vi "PH_Cont-601k_PSU.PC Set Interlock.vi"(0 "VI in":refnum<vi>, 2 "Set Interlock":bool, 5 "error in (no error)":errorcluster) -> (14 "VI out":refnum<vi>, 19 "error out":errorcluster)   [LabVIEW 2014, in "PH_Cont-601k_PSU.lvlib"]
uses:
  PH_Cont-601k_PSU.lvlib
  PH_Cont-601k_PSU.Readyness Program.ctl
  PH_Beckhoff/PH_Beckhoff.lvlib
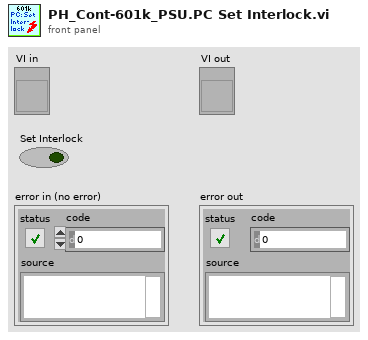
[diagram p1: front panel]
types:
  T1 = typedef "PH_Cont-601k_PSU.lvlib/PH_Cont-601k_PSU.Readyness Program.ctl" = enum32{"OFF", "POWER", "INTERLOCK"}
  T2 = typedef "PH_Cont-601k_PSU.lvlib/PH_Cont-601k_PSU.i attribute.ctl" = cluster{"GUI Refs":T3, "Interlock":bool, "Service ID applied Voltage":i32, "Device Settings":cluster{"Configuration":T4, "Flash Interval [s]":dbl, "Mode":T5, "Voltage [V]":u16, "Charge":bool, "VISA resource name":refnum<visa-resource-name>}, "Readyness":T6, "Information":cluster{"VISA resource name":refnum<visa-resource-name>, "Tagname Power On":string, "Interlock":cluster{"Instance":string, "Tagname":string}, "Limits [V]":cluster{"Lower":dbl, "Upper":dbl}, "Tagname PSU On":string}, "R2S":bool, "Charge is allowed":bool}
  T3 = typedef "PH_Cont-601k_PSU.lvlib/PH_Cont-601k_PSU.GUI Refs.ctl" = cluster{"Power On":refnum<vi>, "Hard- and Software":refnum<vi>, "Device Status":refnum<vi>, "Device Error":refnum<vi>, "Configuration":refnum<vi>, "Flash Interval [s]":refnum<vi>, "Interlock":refnum<vi>, "Interlock Indicator":refnum<vi>, "Voltage [V]":refnum<vi>, "Readyness":refnum<vi>, "Mode":refnum<vi>, "Reset Error":refnum<vi>, "Expert working":refnum<vi>, "Charge":refnum<vi>, "PSU On":refnum<vi>}
  T4 = typedef "PH_Cont-601k_PSU.lvlib/PH_Cont-601k_PSU.Configuration.ctl" = u16
  T5 = typedef "PH_Cont-601k_PSU.lvlib/PH_Cont-601k_PSU.Mode.ctl" = enum32{"STOP", "STANDBY", "READY", "EMISSION", "ERROR"}
  T6 = typedef "PH_Cont-601k_PSU.lvlib/PH_Cont-601k_PSU.Readyness.ctl" = cluster{"Program":T1, "Device":T7}
  T7 = typedef "PH_Cont-601k_PSU.lvlib/PH_Cont-601k_PSU.Readyness Device.ctl" = enum32{"OFF", "CONNECTING", "CONNECTED", "OPERATING", "EOC", "ERROR"}
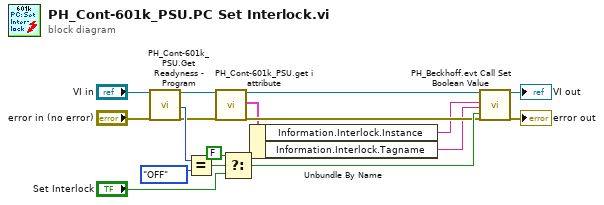
[diagram p0: block diagram]
diagram:
  n1 = call "PH_Cont-601k_PSU.Get Readyness - Program.vi"("VI in"="VI in", "error in (no error)"="error in (no error)") -> ("VI out"=w9:refnum<vi>, "Readyness - Programm"=w12:T1, "error out"=w11:errorcluster)  [unwired: 15 in]
  n2 = Equal?(x=w12, y=PH_Cont-601k_PSU.Readyness_Program."OFF" ("Readyness - Programm")) -> (x = y?=w14:bool)
  n3 = call "PH_Cont-601k_PSU.get i attribute.vi"("i ref in"=w9, "error in (no error)"=w11) -> ("i ref out"=w7:refnum<vi>, "i attribute"=w3:T2, "error out"=w6:errorcluster)  [unwired: 15 in]
  n4 = Select(t=FALSE, s=w14, f="Set Interlock") -> (s? t:f=w16:bool)
  n5 = Unbundle By Name(w3) -> ("Information.Interlock.Instance"=w2:string, "Information.Interlock.Tagname"=w1:string)
  n6 = call "PH_Beckhoff.evt Call Set Boolean Value.vi"("i ref in"=w7, "Beckhoff Instance"=w2, "Tagname to set"=w1, "Value"=w16, "error in"=w6) -> ("i ref out"=→"VI out":refnum<vi>, "error out"=→"error out":errorcluster)  [unwired: 13 in]
